vi "DetectCamera.vi"(8 "error in (no error)":errorcluster, 11 "Config In":T1) -> (0 "error out":errorcluster, 3 "Config Out":T1)   [LabVIEW 2019]
uses:
  Settings/Settings.ctl
  Support/Hardware Configuration.ctl
  Support/Camera Configuration.ctl
  E:/DevHardSoftware/MMicroscopy/HardwareAdapter/Camera/Dependencies/PVCamNET.dll
  Dependencies/PVCamNET.dll
  <vilib>/userdefined/High Color/IMAQdx.ctl
  Logging/Logging Configuration.ctl
  controls/UI Configuration.ctl
  Logging/Logging.lvlib
  Settings/Settings.lvlib
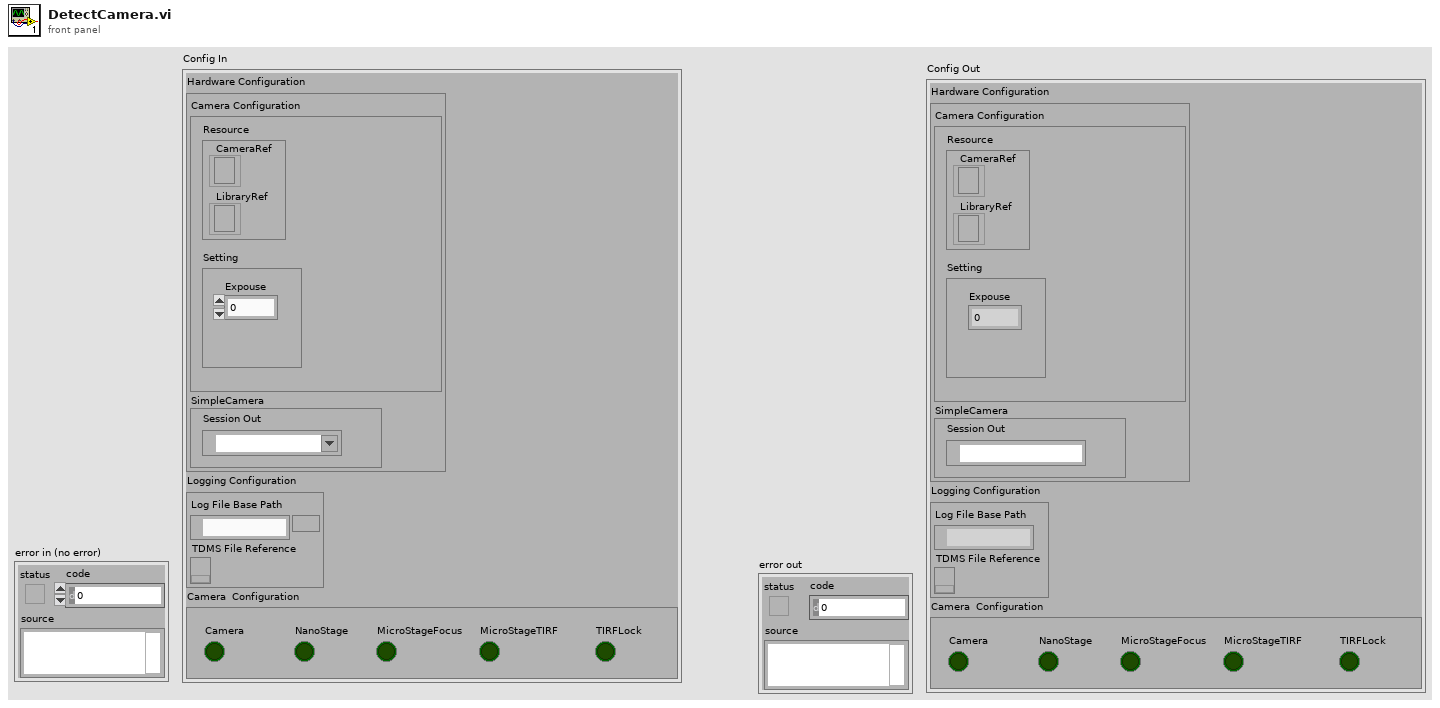
[diagram p1: front panel]
types:
  T1 = typedef "Settings.lvlib/Settings.ctl" = cluster{"Hardware Configuration":T2, "Logging Configuration":T5, "UI Configuration":T6}
  T2 = typedef "Hardware Configuration.ctl" = cluster{"Camera Configuration":T3, "SimpleCamera":cluster{"Session Out":T4}}
  T3 = typedef "Camera Configuration.ctl" = cluster{"Resource":cluster{"CameraRef":refnum<k24>, "LibraryRef":refnum<k24>}, "Setting":cluster{"Expouse":dbl}}
  T4 = typedef "IMAQdx.ctl" = refnum<k21>
  T5 = typedef "Logging.lvlib/Logging Configuration.ctl" = cluster{"Log File Base Path":path, "TDMS File Reference":refnum<k34>}
  T6 = typedef "UI Configuration.ctl" = cluster{"Camera":bool, "NanoStage":bool, "MicroStageFocus":bool, "MicroStageTIRF":bool, "TIRFLock":bool}
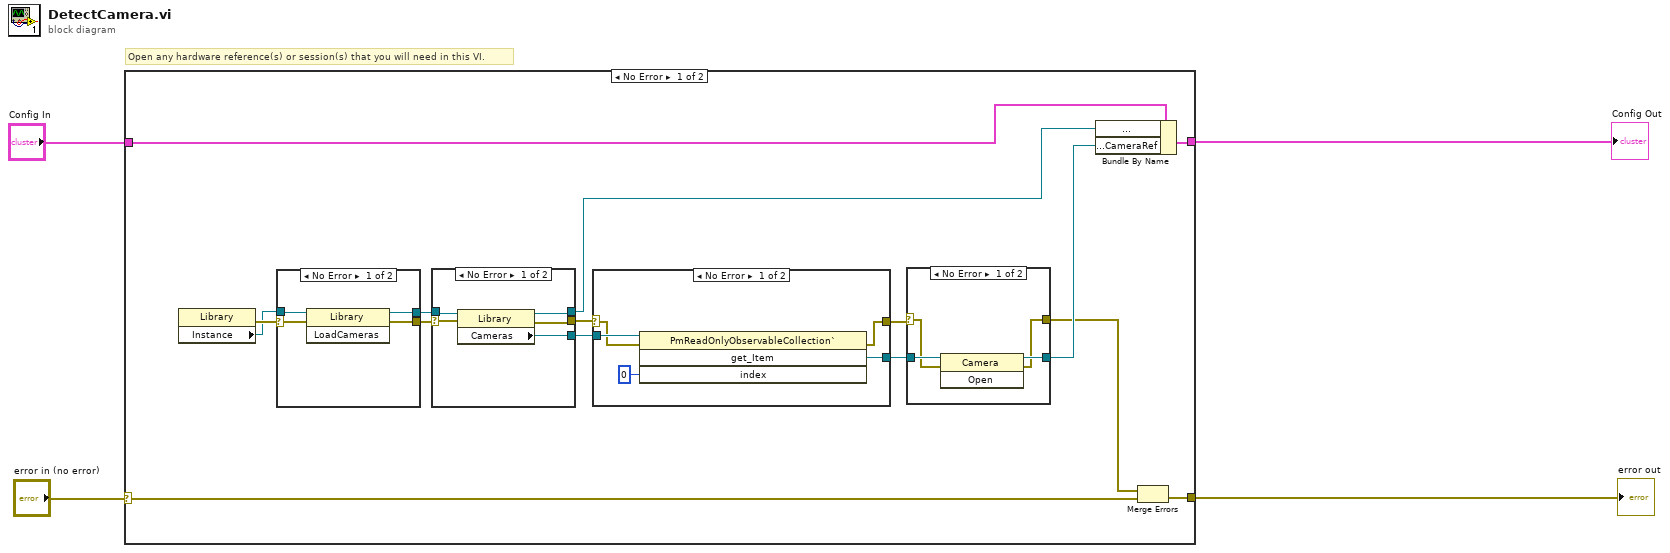
[diagram p0: block diagram]
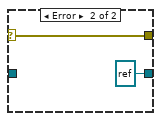
[diagram p2: hidden frame]
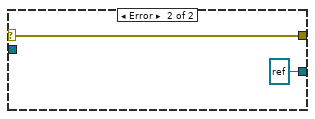
[diagram p3: hidden frame]
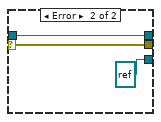
[diagram p4: hidden frame]
diagram:
  # "Open any hardware reference(s) or session(s) that you will need in this VI."
  n1 = case shown="No Error" "error in (no error)" {
    selector: "error in (no error)" -> [w19 w47]
    tunnel: [w18 w47] -> w3
    tunnel: "Config In" -> [w9 w48]
    tunnel: [w8 w48] -> w1
    frame No Error {
      n2 = property class="Library"() -> (error out=w17:errorcluster, "Instance"=w14:refnum<k24>)  [unwired: 2 in, 1 out]
      n3 = case shown="No Error" w17 {
        selector: w17 -> [w42 w46]
        tunnel: [w43 w46] -> w15
        tunnel: [w44 w45] -> w16
        tunnel: w14 -> [w41 w45]
        frame No Error {
          n4 = invoke class="Library" method="LoadCameras"(reference=w41, error in=w42) -> (reference out=w44:refnum<k24>, error out=w43:errorcluster)  [unwired: 1 in, 1 out]
        }
        frame Error {
        }
      }
      n5 = case shown="No Error" w15 {
        selector: w15 -> [w37 w40]
        tunnel: [w34 w40] -> w11
        tunnel: w16 -> [w36 w39]
        tunnel: [w35 w39] -> w7
        tunnel: [w33 refnum<k24> refnum ("Cameras")] -> w13
        frame No Error {
          n6 = property class="Library"(reference=w36, error in=w37) -> (reference out=w35:refnum<k24>, error out=w34:errorcluster, "Cameras"=w33:refnum<k24>)
        }
        frame Error {
        }
      }
      n7 = case shown="No Error" w11 {
        selector: w11 -> [w27 w32]
        tunnel: w13 -> [w30 _]
        tunnel: [w28 refnum<k24> refnum ("get_Item")] -> w12
        tunnel: [w26 w32] -> w10
        frame No Error {
          n8 = invoke class="PmReadOnlyObservableCollection`" method="get_Item"(reference=w30, error in=w27, "index"=0) -> (error out=w26:errorcluster, "get_Item"=w28:refnum<k24>)  [unwired: 1 in, 2 out]
        }
        frame Error {
        }
      }
      n9 = case shown="No Error" w10 {
        selector: w10 -> [w21 w25]
        tunnel: [w20 w25] -> w5
        tunnel: w12 -> [w23 _]
        tunnel: [w22 refnum<k24> refnum ("get_Item")] -> w6
        frame No Error {
          n10 = invoke class="Camera" method="Open"(reference=w23, error in=w21) -> (reference out=w22:refnum<k24>, error out=w20:errorcluster)  [unwired: 1 in, 1 out]
        }
        frame Error {
        }
      }
      n11 = Bundle By Name(cluster=w9, "Hardware Configuration.Camera Configuration.Resource.LibraryRef"=w7, "Hardware Configuration.Camera Configuration.Resource.CameraRef"=w6) -> (w8:T1)
      n12 = Merge Errors(w5, w19) -> (w18:errorcluster)
    }
    frame Error {
    }
  }
  "error out" <- w3
  "Config Out" <- w1
